vi "Pane.vi"(6 "Selection Colors":T1={"Normal"=13816530, "Mouse-over"=0, "Selected"=9868950, "Selected Mouse-over"=9868950}, 7 "Settings UI Enqueuer":refnum<class "Message Enqueuer.lvclass">, 8 "Error In":errorcluster, 9 "Offset":T2, 10 "Scale Factor":dbl, 11 "Pane Ref":refnum<vi>) -> (0 "Error Out":errorcluster, 3 "Pane out":refnum<class "Pane.lvclass">)   [LabVIEW 2018, in "Pane.lvclass"]
uses:
  <resource>/dialog/QuickDrop/plugins/PaneRelief/Classes/Pane/Pane.lvclass
  C:/Program Files (x86)/National Instruments/LabVIEW 2018/resource/dialog/QuickDrop/plugins/PaneRelief/Classes/Panel Object/Panel Object.lvclass
  <resource>/dialog/QuickDrop/plugins/PaneRelief/Typedefs/Point--Cluster.ctl
  <vilib>/ActorFramework/Message Enqueuer/Message Enqueuer.lvclass
  <resource>/dialog/QuickDrop/plugins/PaneRelief/Typedefs/Selection Colors--Cluster.ctl
  <resource>/dialog/QuickDrop/plugins/PaneRelief/Typedefs/Rectangle--Cluster.ctl
  <resource>/dialog/QuickDrop/plugins/PaneRelief/Classes/Panel Object/Panel Object.lvclass/Panel Object.ctl
  <resource>/dialog/QuickDrop/plugins/PaneRelief/Classes/Pane/Pane.lvclass/Pane.ctl
  <resource>/dialog/QuickDrop/plugins/PaneRelief/Classes/Panel Object/Write Bounds.vi
  <resource>/dialog/QuickDrop/plugins/PaneRelief/Classes/Panel Object/Write Settings UI Enqueuer.vi
  <resource>/dialog/QuickDrop/plugins/PaneRelief/Classes/Panel Object/Write Selection Colors.vi
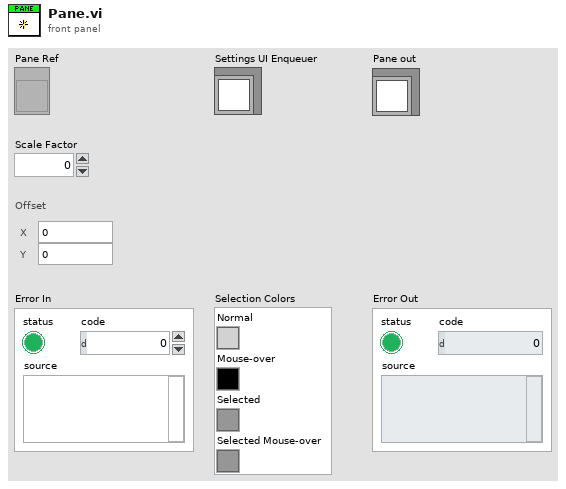
[diagram p1: front panel]
types:
  T1 = typedef "Selection Colors--Cluster.ctl" = cluster{"Normal":u32, "Mouse-over":u32, "Selected":u32, "Selected Mouse-over":u32}
  T2 = typedef "Point--Cluster.ctl" = cluster{"Horizontal":i32, "Vertical":i32}
  T3 = typedef "Rectangle--Cluster.ctl" = cluster{"X start":i32, "X end":i32, "Y start":i32, "Y end":i32}
  T4 = typedef "LVPointTypeDef.ctl" = cluster{"Horizontal":i16, "Vertical":i16}
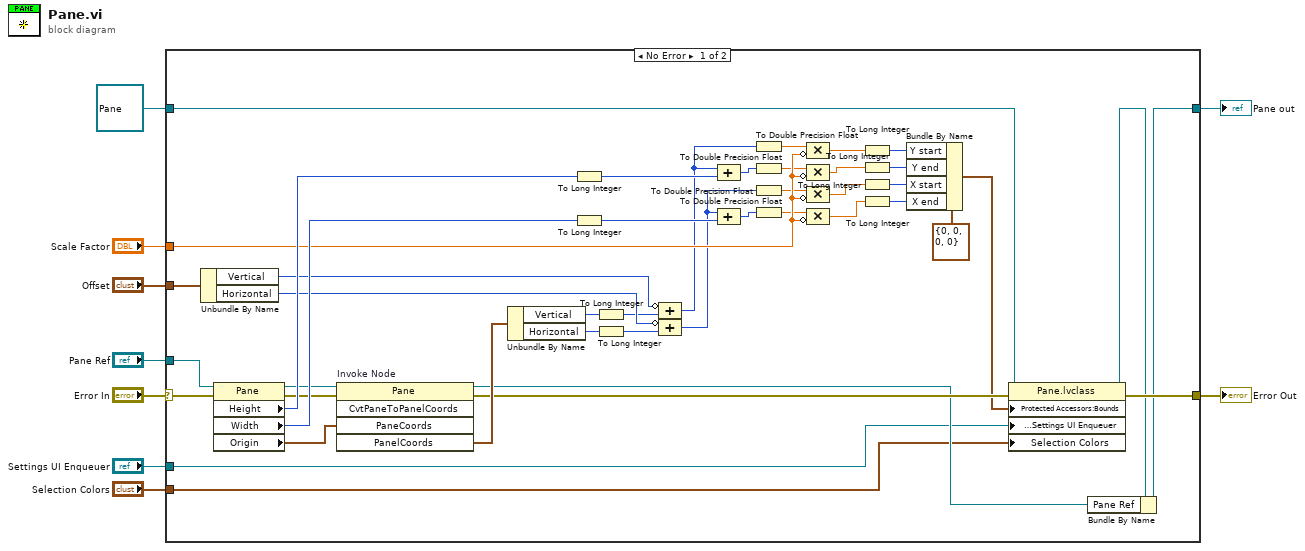
[diagram p0: block diagram]
diagram:
  n1 = case shown="No Error" "Error In" {
    selector: "Error In" -> [w37 w55]
    tunnel: [w24 w55] -> w7
    tunnel: [w19 w54] -> w9
    tunnel: refnum<class "Pane.lvclass"> refnum ("Pane in") -> [w21 w54]
    tunnel: "Offset" -> [w38 _]
    tunnel: "Pane Ref" -> [w36 _]
    tunnel: "Scale Factor" -> [w35 _]
    tunnel: "Settings UI Enqueuer" -> [w11 _]
    tunnel: "Selection Colors" -> [w10 _]
    frame No Error {
      n2 = Unbundle By Name(w38) -> ("Vertical"=w12:i32, "Horizontal"=w15:i32)
      n3 = property class="Pane"(reference=w36, error in=w37) -> (reference out=w49:refnum<vi>, error out=w48:errorcluster, "Height"=w53:u32, "Width"=w52:u32, "Origin"=w34:T4)
      n4 = invoke on="Invoke Node" class="Pane" method="CvtPaneToPanelCoords"(reference=w49, error in=w48, "PaneCoords"=w34) -> (reference out=w18:refnum<vi>, error out=w25:errorcluster, "PanelCoords"=w47:T4)  [unwired: 2 in, 2 out]
      n5 = Unbundle By Name(w47) -> ("Vertical"=w40:i16, "Horizontal"=w39:i16)
      n6 = To Long Integer(number=w53) -> (32bit integer=w42:i32)
      n7 = To Long Integer(number=w52) -> (32bit integer=w41:i32)
      n8 = To Long Integer(number=w40) -> (32bit integer=w14:i32)
      n9 = To Long Integer(number=w39) -> (32bit integer=w17:i32)
      n10 = Compound Arithmetic op=ADD(invert w12, w14) -> (w13:i32)
      n11 = Compound Arithmetic op=ADD(invert w15, w17) -> (w16:i32)
      n12 = Compound Arithmetic op=ADD(w13, w42) -> (w51:i32)
      n13 = Compound Arithmetic op=ADD(w16, w41) -> (w50:i32)
      n14 = To Double Precision Float(number=w13) -> (double precision float=w29:dbl)
      n15 = To Double Precision Float(number=w51) -> (double precision float=w28:dbl)
      n16 = To Double Precision Float(number=w16) -> (double precision float=w27:dbl)
      n17 = To Double Precision Float(number=w50) -> (double precision float=w26:dbl)
      n18 = Compound Arithmetic op=MULTIPLY(w29, invert w35) -> (w45:dbl)
      n19 = Compound Arithmetic op=MULTIPLY(w28, invert w35) -> (w44:dbl)
      n20 = Compound Arithmetic op=MULTIPLY(w27, invert w35) -> (w43:dbl)
      n21 = Compound Arithmetic op=MULTIPLY(w26, invert w35) -> (w46:dbl)
      n22 = To Long Integer(number=w45) -> (32bit integer=w33:i32)
      n23 = To Long Integer(number=w44) -> (32bit integer=w32:i32)
      n24 = To Long Integer(number=w43) -> (32bit integer=w31:i32)
      n25 = To Long Integer(number=w46) -> (32bit integer=w30:i32)
      n26 = Bundle By Name(cluster=T3 {"X start"=0, "X end"=0, "Y start"=0, "Y end"=0} ("Bounds"), "Y start"=w33, "Y end"=w32, "X start"=w31, "X end"=w30) -> (w22:T3)
      n27 = property class="Pane.lvclass"(reference=w21, error in=w25, "Protected Accessors:Bounds"=w22, "Protected Accessors:Settings UI Enqueuer"=w11, "Selection Colors"=w10) -> (reference out=w20:refnum<class "Pane.lvclass">, error out=w24:errorcluster)
      n28 = Bundle By Name(cluster=w20, "Pane Ref"=w18) -> (w19:refnum<class "Pane.lvclass">)
    }
    frame Error {
    }
  }
  "Pane out" <- w9
  "Error Out" <- w7
